vi "Test Q calca.vi"() -> ()   [LabVIEW 2012]
panel:
  out "max":dbl
  out "Q with offset":dbl
  out "width with offset":dbl
  out "w3":dbl
  out "width with no offset":dbl
  out "Q3":dbl
  out "Q no offset":dbl
  out "Q1":dbl
  out "x+y":i32[](array[numeric])
  out "Array":dbl[](array[numeric])
  out "XY Graph":cluster{i32[], dbl[]}(graph)
  in  "a":dbl[](array[numeric])
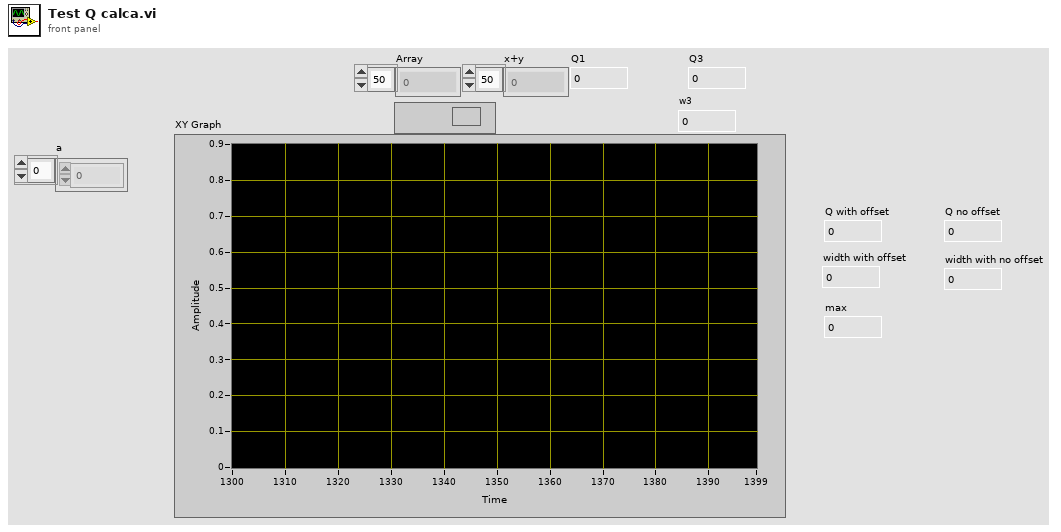
[diagram p1: front panel]
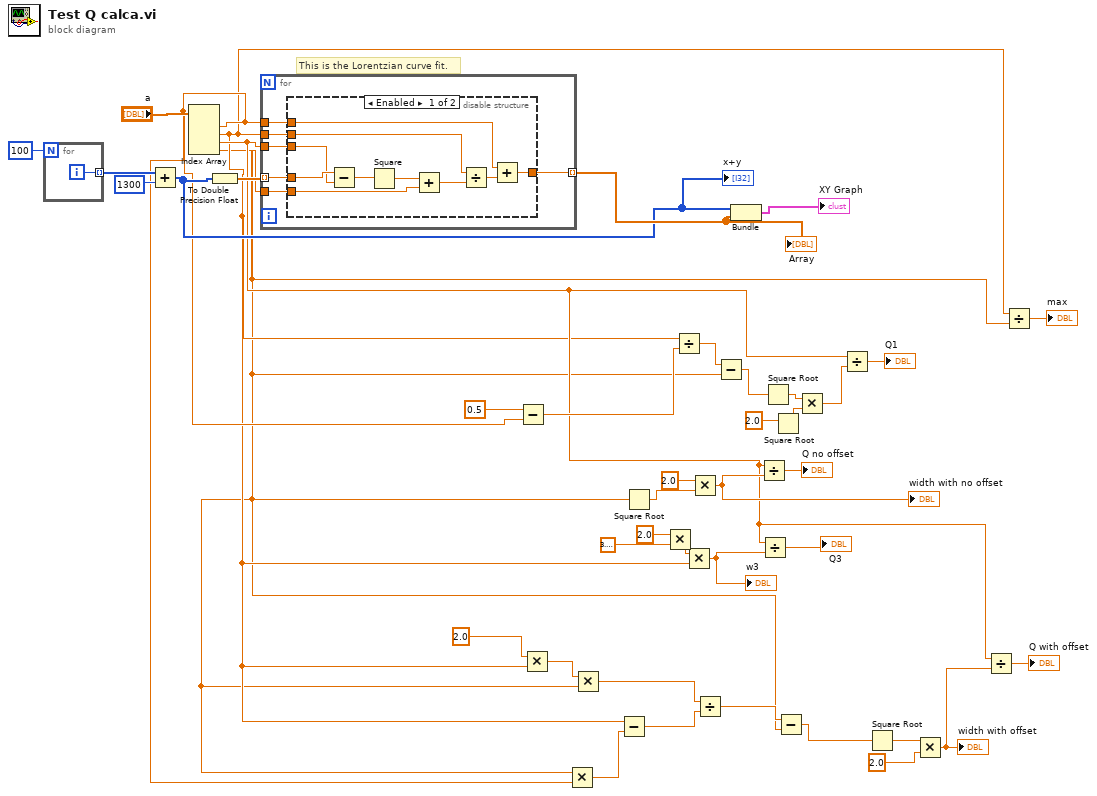
[diagram p0: block diagram]
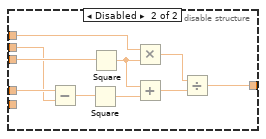
[diagram p2: hidden frame]
diagram:
  # "This is the Lorentzian curve fit."
  n1 = for {
    N: 100 -> [_]
    tunnel: [w43] -> w39 mode=indexing
    i -> [w43]
  }
  n2 = Add(x=w39, y=1300) -> (x+y=w19:i32[])
  "x+y" <- w19
  n3 = Index Array(array="a") -> (element #1=w14:dbl, element #2=w3:dbl, element #3=w5:dbl, element #4=w2:dbl)  [unwired: 4 in]
  n4 = To Double Precision Float(number=w19) -> (double precision float=w37:dbl[])
  n5 = for {
    tunnel: w37 -> [w49] mode=indexing
    tunnel: w14 -> [w48]
    tunnel: w3 -> [w46]
    tunnel: w5 -> [w47]
    tunnel: w2 -> [w45]
    tunnel: [w44] -> w20 mode=indexing
    n6 = disable-structure shown="Enabled" {
      disable-tunnel: w49 -> [w59 w66]
      disable-tunnel: w48 -> [w57 w69]
      disable-tunnel: w47 -> [w56 w68]
      disable-tunnel: w46 -> [w55 w65]
      disable-tunnel: w45 -> [w54 _]
      disable-tunnel: [w50 w60] -> w44
      frame Enabled {
        n7 = Subtract(x=w59, y=w56) -> (x-y=w58:dbl)
        n8 = Square(x=w58) -> (x^2=w53:dbl)
        n9 = Add(x=w53, y=w54) -> (x+y=w52:dbl)
        n10 = Divide(x=w55, y=w52) -> (x/y=w51:dbl)
        n11 = Add(x=w57, y=w51) -> (x+y=w50:dbl)
      }
      frame Disabled {
        n12 = Subtract(x=w66, y=w65) -> (x-y=w64:dbl)
        n13 = Square(x=w64) -> (x^2=w62:dbl)
        n14 = Square(x=w68) -> (x^2=w63:dbl)
        n15 = Multiply(x=w69, y=w63) -> (x*y=w67:dbl)
        n16 = Add(x=w63, y=w62) -> (x+y=w61:dbl)
        n17 = Divide(x=w67, y=w61) -> (x/y=w60:dbl)
      }
    }
  }
  "Array" <- w20
  n18 = Subtract(x=0.5 ("y"), y=w14) -> (x-y=w21:dbl)
  n19 = Multiply(x=2.0, y=w3) -> (x*y=w15:dbl)
  n20 = Multiply(x=w2, y=w14) -> (x*y=w13:dbl)
  n21 = Multiply(x=w15, y=w2) -> (x*y=w12:dbl)
  n22 = Subtract(x=w3, y=w13) -> (x-y=w11:dbl)
  n23 = Square Root(x=w2) -> (sqrt(x)=w32:dbl)
  n24 = Multiply(x=2.0, y=3.141592653589793) -> (x*y=w25:dbl)
  n25 = Divide(x=w3, y=w21) -> (x/y=w36:dbl)
  n26 = Multiply(x=w25, y=w3) -> (x*y=w24:dbl)
  "w3" <- w24
  n27 = Multiply(x=2.0, y=w32) -> (x*y=w30:dbl)
  "width with no offset" <- w30
  n28 = Divide(x=w12, y=w11) -> (x/y=w10:dbl)
  n29 = Subtract(x=w36, y=w2) -> (x-y=w35:dbl)
  n30 = Bundle(w19, w20) -> (→"XY Graph":cluster{i32[], dbl[]})  [unwired: 1 in]
  n31 = Divide(x=w5, y=w30) -> (x/y=→"Q no offset":dbl)
  n32 = Divide(x=w5, y=w24) -> (x/y=→"Q3":dbl)
  n33 = Square Root(x=w35) -> (sqrt(x)=w34:dbl)
  n34 = Square Root(x=2.0 ("y")) -> (sqrt(x)=w17:dbl)
  n35 = Subtract(x=w10, y=w2) -> (x-y=w9:dbl)
  n36 = Multiply(x=w34, y=w17) -> (x*y=w29:dbl)
  n37 = Divide(x=w5, y=w29) -> (x/y=→"Q1":dbl)
  n38 = Square Root(x=w9) -> (sqrt(x)=w8:dbl)
  n39 = Multiply(x=w8, y=2.0 ("x")) -> (x*y=w6:dbl)
  "width with offset" <- w6
  n40 = Divide(x=w5, y=w6) -> (x/y=→"Q with offset":dbl)
  n41 = Divide(x=w3, y=w2) -> (x/y=→"max":dbl)
